vi "BoltzmannConstant.vi"() -> ()   [LabVIEW 2012]
panel:
  in  "Intrinsic Noise":dbl
  in  "Temperature (K)":dbl
  in  "Resistance (Ohms)":dbl
  in  "Gain":dbl
  out "Waveform Chart 2":dbl(graph)
  out "Waveform Chart":dbl(graph)
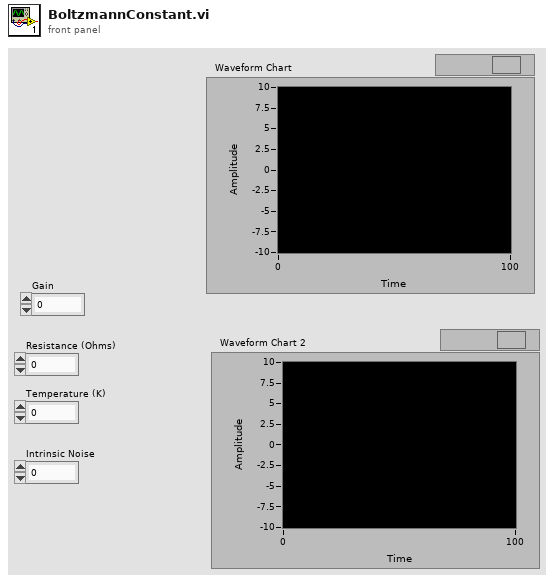
[diagram p1: front panel]
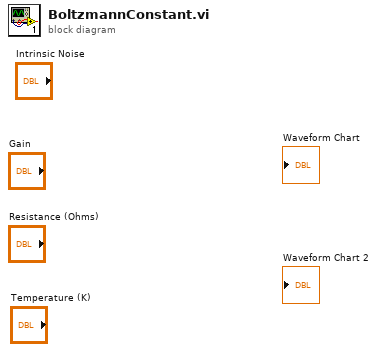
[diagram p0: block diagram]
diagram:
